vi "Update Title.vi"(0 "Room Service Manager UI in":refnum<class "Room Service Manager UI.lvclass">, 5 "Room No":string, 11 "error in (no error)":errorcluster) -> (4 "Room Service Manager UI out":refnum<class "Room Service Manager UI.lvclass">, 15 "error out":errorcluster)   [LabVIEW 2023, in "Room Service Manager UI.lvlib" / "Room Service Manager UI.lvclass"]
uses:
  Room Service Manager UI.lvclass
  Room Service Manager UI.lvclass/Room Service Manager UI.ctl
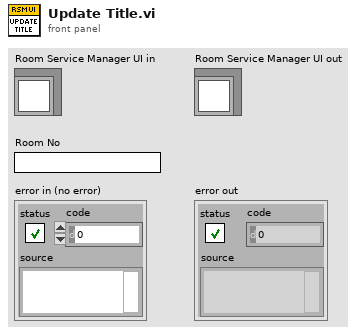
[diagram p1: front panel]
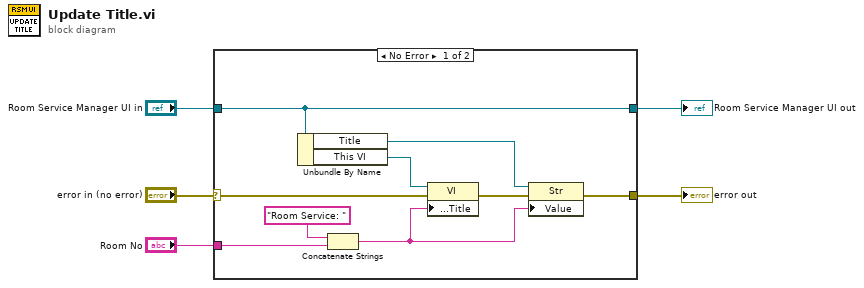
[diagram p0: block diagram]
diagram:
  n1 = case shown="No Error" "error in (no error)" {
    selector: "error in (no error)" -> [w14 w16]
    tunnel: [w9 w16] -> w4
    tunnel: [w13 w15] -> w2
    tunnel: "Room Service Manager UI in" -> [w13 w15]
    tunnel: "Room No" -> [w8 _]
    frame No Error {
      n2 = Unbundle By Name(w13) -> ("Title"=w10:refnum<vi>, "This VI"=w12:refnum<vi>)
      n3 = Concatenate Strings("Room Service: " ("string"), w8) -> (w6:string)
      n4 = property class="VI"(reference=w12, error in=w14, "Front Panel.Title"=w6) -> (error out=w11:errorcluster)  [unwired: 1 out]
      n5 = property class="Str"(reference=w10, error in=w11, "Value"=w6) -> (error out=w9:errorcluster)  [unwired: 1 out]
    }
    frame Error {
    }
  }
  "error out" <- w4
  "Room Service Manager UI out" <- w2
